vi "SetStrToStrCtrl.vi"(10 "Value":string, 11 "ref str in":refnum<vi>) -> ()   [LabVIEW 2018, in "Library-Ctrl.lvlib"]
uses:
  Library-Ctrl.lvlib
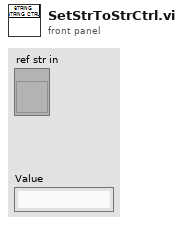
[diagram p1: front panel]
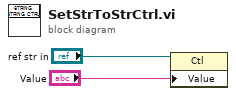
[diagram p0: block diagram]
diagram:
  n1 = property class="Ctl"(reference="ref str in", "Value"="Value") -> ()  [unwired: 1 in, 2 out]
